vi "test.vi"() -> ()   [LabVIEW 2015]
panel:
  in  "2":bool
  in  "1":bool
  in  "0":bool=TRUE
  out "number 2":u32
  out "element 8":bool
  out "element 7":bool
  out "element 6":bool
  out "element 5":bool
  out "element 4":bool
  out "element 3":bool
  out "element 2":bool
  out "element":bool
  in  "number":u8
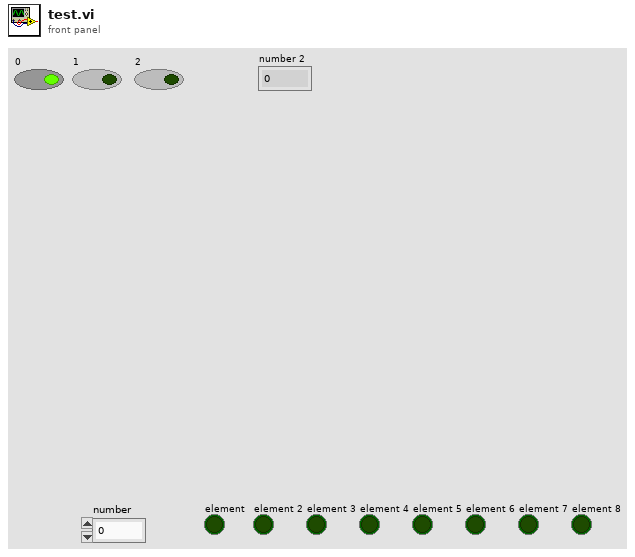
[diagram p1: front panel]
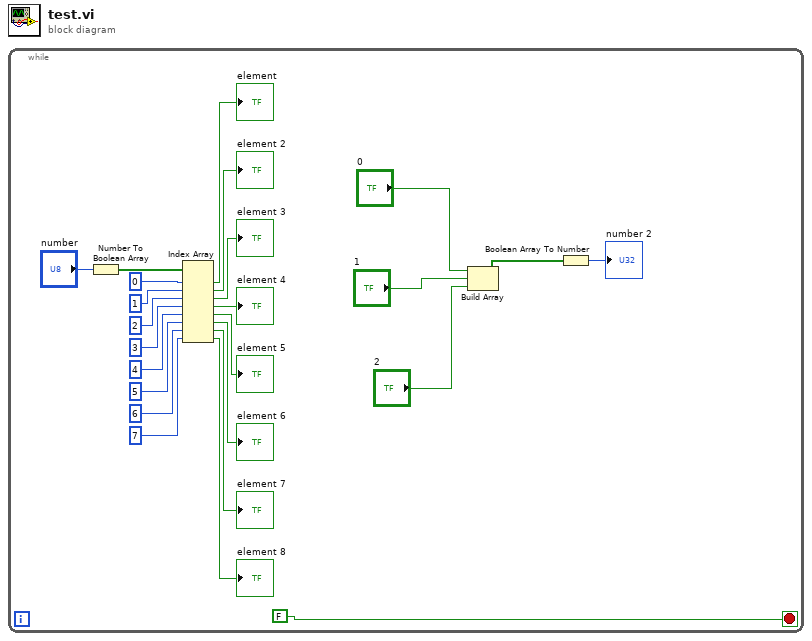
[diagram p0: block diagram]
diagram:
  n1 = while {
    stop <- FALSE stop-if-true
    n2 = Number To Boolean Array(number="number") -> (Boolean array=w15:bool[])
    n3 = Index Array(array=w15, index #1=0 ("index"), index #2=1 ("index"), index #3=2 ("index"), index #4=3 ("index"), index #5=4 ("index"), index #6=5 ("index"), index #7=6 ("index"), index #8=7 ("index")) -> (element #1=→"element":bool, element #2=→"element 2":bool, element #3=→"element 3":bool, element #4=→"element 4":bool, element #5=→"element 5":bool, element #6=→"element 6":bool, element #7=→"element 7":bool, element #8=→"element 8":bool)
    n4 = Build Array("0", "1", "2") -> (w3:bool[])
    n5 = Boolean Array To Number(Boolean array=w3) -> (number=→"number 2":u32)
  }
